vi "Delete.vi"(8 "error in (no error)":errorcluster, 10 "Index":i32, 11 "Assembly In":refnum<class "Assembly Run.lvclass">) -> (0 "error out":errorcluster, 3 "Assembly Out":refnum<class "Assembly Run.lvclass">)   [LabVIEW 2016, in "Assembly Run.lvclass"]
uses:
  Assembly Run.lvclass
  Assembly Run.lvclass/Assembly Run.ctl
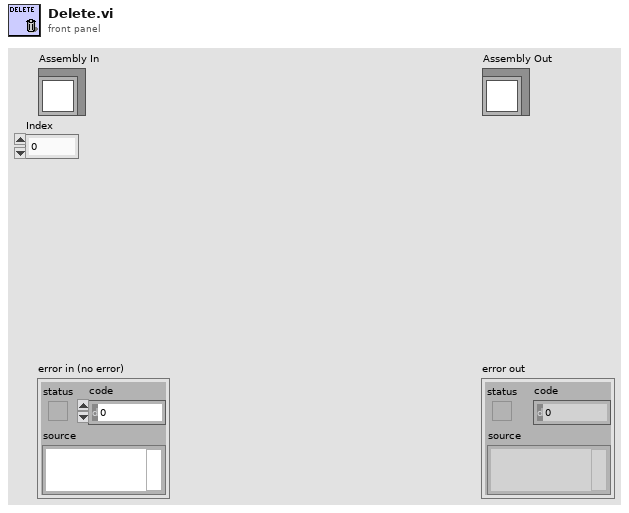
[diagram p1: front panel]
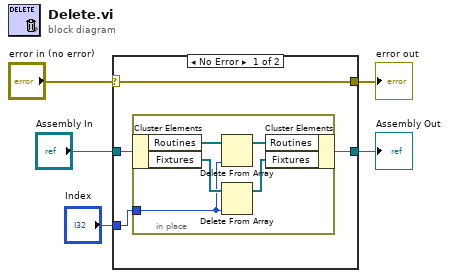
[diagram p0: block diagram]
diagram:
  n1 = case shown="No Error" "error in (no error)" {
    selector: "error in (no error)" -> [w9 w16]
    tunnel: [w9 w16] -> w4
    tunnel: [w6 w15] -> w2
    tunnel: "Assembly In" -> [w7 w15]
    tunnel: "Index" -> [w8 _]
    frame No Error {
      n2 = in-place {
        in-place-border: w8 -> [w12]
        n3 = in-place-cluster #1(w7) -> ("Routines"=w14:refnum<class "Routine.lvclass">[], "Fixtures"=w13:refnum<class "Fixture.lvclass">[])
        n4 = Delete From Array(array=w14, index=w12) -> (array with subset deleted=w11:refnum<class "Routine.lvclass">[])  [unwired: 1 in, 1 out]
        n5 = Delete From Array(array=w13, index=w12) -> (array with subset deleted=w10:refnum<class "Fixture.lvclass">[])  [unwired: 1 in, 1 out]
        n6 = in-place-cluster #1("Routines"=w11, "Fixtures"=w10) -> (w6:refnum<class "Assembly Run.lvclass">)
      }
    }
    frame Error {
    }
  }
  "error out" <- w4
  "Assembly Out" <- w2
